vi "Evaluation_peak.vi"(1 "X2":sgl=inf, 2 "X1":sgl=-inf, 3 "Data":cluster{dbl[], dbl[]}) -> (0 "Area":sgl format="%0.6e")   [LabVIEW 2010]
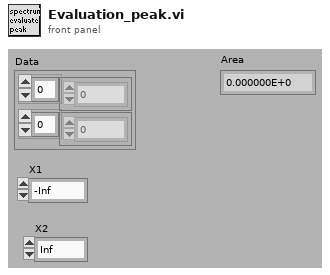
[diagram p1: front panel]
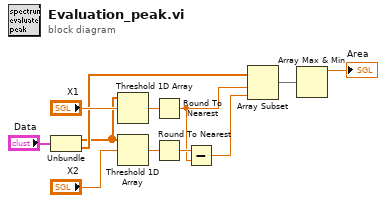
[diagram p0: block diagram]
diagram:
  n1 = Unbundle("Data") -> (w7:dbl[], w9:dbl[])
  n2 = Threshold 1D Array(2:"X1", 3:w7) -> (0:w11:dbl)  [unwired: 1 in]
  n3 = Threshold 1D Array(2:"X2", 3:w7) -> (0:w6:dbl)  [unwired: 1 in]
  n4 = Round To Nearest(number=w11) -> (nearest integer value=w4:dbl)
  n5 = Round To Nearest(number=w6) -> (nearest integer value=w5:dbl)
  n6 = Subtract(x=w5, y=w4) -> (x-y=w3:dbl)
  n7 = Array Subset(array=w9, index=w4, length=w3) -> (w2:dbl[])
  n8 = Array Max & Min(array=w2) -> (max value=→"Area":dbl)  [unwired: 3 out]
